vi "ProcessModbusUpdates.vi"(11 "MockHPILCSettings":T1={"ModbusRxDataFIFO"="MockbusPort2RxFIFO", "ModbusTxDataFIFO"="MockbusPort2TxFIFO", "BufferUpdateFIFO"="MockHPILCCommand", "Code17Memory"="MockHPILCCode17", "Code18Memory"="MockHPILCCode18", "Code65Memory"="MockHPILCCode65", "Code66Memory"="MockHPILCCode66", "Code67Memory"="MockHPILCCode67", "Code72Memory"="MockHPILCCode72", "Code80Memory"="MockHPILCCode80", "Code110Memory"="MockHPILCCode110", "CRCDataFIFO"="MockHPILCCRCDataFIFO", "CRCCalculateFIFO"="MockHPILCCRCCalculateFIFO", "CRCFIFO"="MockHPILCCRCFIFO"}) -> ()   [LabVIEW 2016, in "FPGAMockHPILC.lvlib"]
uses:
  FPGAMockHPILC.lvlib
  DataTypes/MockHPILCSettings.ctl
  DataTypes/MockHPModbusUpdateLoopData.ctl
  DataTypes/MockHPModbusUpdateStates.ctl
  <vilib>/Platform/TimedLoop/XDataNode/timing_clust.ctl
  <vilib>/Platform/TimedLoop/XDataNode/nitl_modes.ctl
  <vilib>/Platform/TimedLoop/XDataNode/wakeup.ctl
  <vilib>/rvi/Emulation/niFpgaSctlEmulationGetInTimedLoop.vi
  <vilib>/rvi/Emulation/niFpgaEmulationReportErrorSimple.vi
  <vilib>/rvi/Emulation/niFpgaGetClockAttributes.vi
  <vilib>/rvi/Emulation/niFpgaCriticalErrorInLSC.vi
  <vilib>/rvi/DataTransferAndStorage/Container/Common/niFpgaContainerExecOnDevCompGetState.vi
  <vilib>/rvi/Emulation/niFpgaEmulationIsFPGAContextNoSignature.vi
  <vilib>/rvi/errors/niFpgaSetErrorForExecOnDevCompSimple.vi
  <vilib>/rvi/eio/common/nirviEmuReportErrorAndStop.vi
  <vilib>/rvi/DataTransferAndStorage/Container/Common/niFpgaContainerGetUniqueNameForEmu.vi
  <vilib>/rvi/FIFO/Fifo_Resource/nirvififoEmulationSetSize.vi
  <vilib>/rvi/FIFO/Fifo_Resource/nirviFifoEmulationQueueMgr.vi
  <instcachedir>/0/nirviFifoEmulationQueueMgr_E5CAEC123FF24DC58D834DCA3CDAA9B5.lvgen/nirviFifoEmulationQueueMgr_E5CAEC123FF24DC58D834DCA3CDAA9B5_002.vi
  <vilib>/rvi/FIFO/Fifo_Resource/nirvififoEmulationDetermineInputValidOut.vi
  <vilib>/rvi/FIFO/Fifo_Resource/nirvififoEmulationCreateLock.vi
  <vilib>/rvi/Emulation/niFpgaProcessEmulError.vi
  <vilib>/rvi/FIFO/Fifo_Resource/nirvififoEmulationObtainLock.vi
  <vilib>/rvi/FIFO/Fifo_Resource/nirvififoEmulationReleaseLock.vi
  <vilib>/rvi/occurrence/nirviWaitOnOccurrenceBase.vi
  <vilib>/rvi/errors/nirviReportUnexpectedCaseInternalError.vi
  <vilib>/rvi/errors/nirviReportUnexpectedCaseInternalError (U32).vi
  <vilib>/Utility/error.llb/Clear Errors.vi
  <vilib>/rvi/interface/RandomDataEmulation/niFpgaRandomDataHandleErrors.vi
  <instcachedir>/0/nirviFifoEmulationQueueMgr_E5CAEC123FF24DC58D834DCA3CDAA9B5.lvgen/nirviFifoEmulationQueueMgr_E5CAEC123FF24DC58D834DCA3CDAA9B5_009.vi
  <vilib>/rvi/Memory/Memory_Emulation/niFpgaMemoryEmulationCacheClearOnFirstRun.vi
  <vilib>/rvi/Memory/Memory_Emulation/nirvimemoryEmulationManagerCache_MakeExclusive.vi
  <vilib>/rvi/Memory/Memory_Emulation/niFpgaMemoryEmulationValidateCache.vi
  <vilib>/rvi/Memory/Memory_Emulation/nirvimemoryEmulationManagerCache_InsertValue.vi
  <vilib>/rvi/Memory/Memory_Emulation/nirvimemoryEmulationManagerCache_ReleaseExclusive.vi
  <vilib>/rvi/Memory/Memory_Emulation/nirvimemoryEmulationManagerCache_GetValue.vi
  <vilib>/rvi/Memory/Memory_Emulation/nirvimemoryEmulationManagerCache_SetValue.vi
  <vilib>/rvi/Emulation/niFpgaSctlEmulationResourceMgr.vi
  <instcachedir>/0/nirviFifoEmulationQueueMgr_E5CAEC123FF24DC58D834DCA3CDAA9B5.lvgen/nirviFifoEmulationQueueMgr_E5CAEC123FF24DC58D834DCA3CDAA9B5_004.vi
  <vilib>/Platform/TimedLoop/XDataNode/XDataNode.xnode
  <vilib>/rvi/DataTransferAndStorage/Container/XNode/niFpgaContainer.xnode
  <vilib>/rvi/FIFO/Fifo_Resource/niFpgaFifoEmulationRefIn.vi
  <vilib>/rvi/Memory/Memory_Emulation/niFpgaMemoryEmulationRefIn.vi
  <vilib>/Platform/TimedLoop/XDataNode/XDNodeRunTimeDep.lvlib
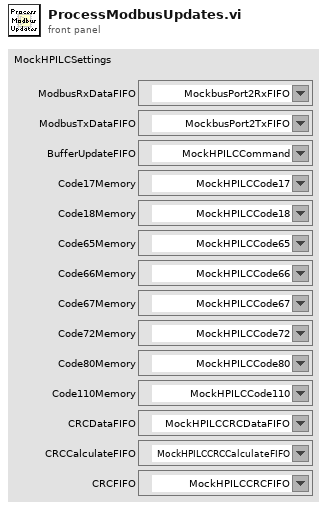
[diagram p1: front panel]
types:
  T1 = typedef "FPGAMockHPILC.lvlib/MockHPILCSettings.ctl" = cluster{"ModbusRxDataFIFO":refnum<k21>, "ModbusTxDataFIFO":refnum<k21>, "BufferUpdateFIFO":refnum<k21>, "Code17Memory":refnum<k21>, "Code18Memory":refnum<k21>, "Code65Memory":refnum<k21>, "Code66Memory":refnum<k21>, "Code67Memory":refnum<k21>, "Code72Memory":refnum<k21>, "Code80Memory":refnum<k21>, "Code110Memory":refnum<k21>, "CRCDataFIFO":refnum<k21>, "CRCCalculateFIFO":refnum<k21>, "CRCFIFO":refnum<k21>}
  T2 = typedef "FPGAMockHPILC.lvlib/MockHPModbusUpdateLoopData.ctl" = cluster{"ModbusUpdateLoopStates":T3, "Address":u8, "Function":u8, "ResponseLength":u8, "ResponseIndex":u8, "Index":u8, "Data":u16, "DelayTicks":u32}
  T3 = typedef "FPGAMockHPILC.lvlib/MockHPModbusUpdateStates.ctl" = enum16{"ReadModbusPort", "ProcessModbusData", "DelayMicroseconds", "WriteAddress", "WriteFunction", "WriteData", "WriteCRCLSB", "WriteCRCMSB", "WriteEndOfFrame", "CalculateCRC"}
  T4 = typedef "XDNodeRunTimeDep.lvlib/timing_clust.ctl" = cluster{"Expected End [f-1]":u64, "Actual End [f-1]":u64, "Finished Late? [f-1]":bool, "Expected End [i-1]":u64, "Actual End [i-1]":u64, "Finished Late? [i-1]":bool, "Expected Start [i]":u64, "Actual Start [i]":u64, "Expected Start [f]":u64, "Actual Start [f]":u64, "Source Name":string, "Structure Name":string, "Period":i64, "Deadline":i64, "Offset":i64, "Start":i64, "Priority":i32, "Timeout":i32, "Mode":T5, "Wakeup Reason":T6, "Error":errorcluster, "Source Type":string, "Secondary Source Type":string, "Global End Time":u64, "Global Start Time":u64, "Frame Duration":u64, "Iteration Duration":u64, "Assigned CPU":i32, "I/O Scan Engine Mode":u32}
  T5 = typedef "XDNodeRunTimeDep.lvlib/nitl_modes.ctl" = enum32{"No Change", "Process missed periods, maintain original phase", "Discard missed periods, maintain original phase", "Process missed periods, ignore original phase", "Discard missed periods, ignore original phase"}
  T6 = typedef "XDNodeRunTimeDep.lvlib/wakeup.ctl" = enum32{"Normal", "Aborted", "Asynchronous wakeup", "Timing source error", "Timed loop error", "Timeout"}
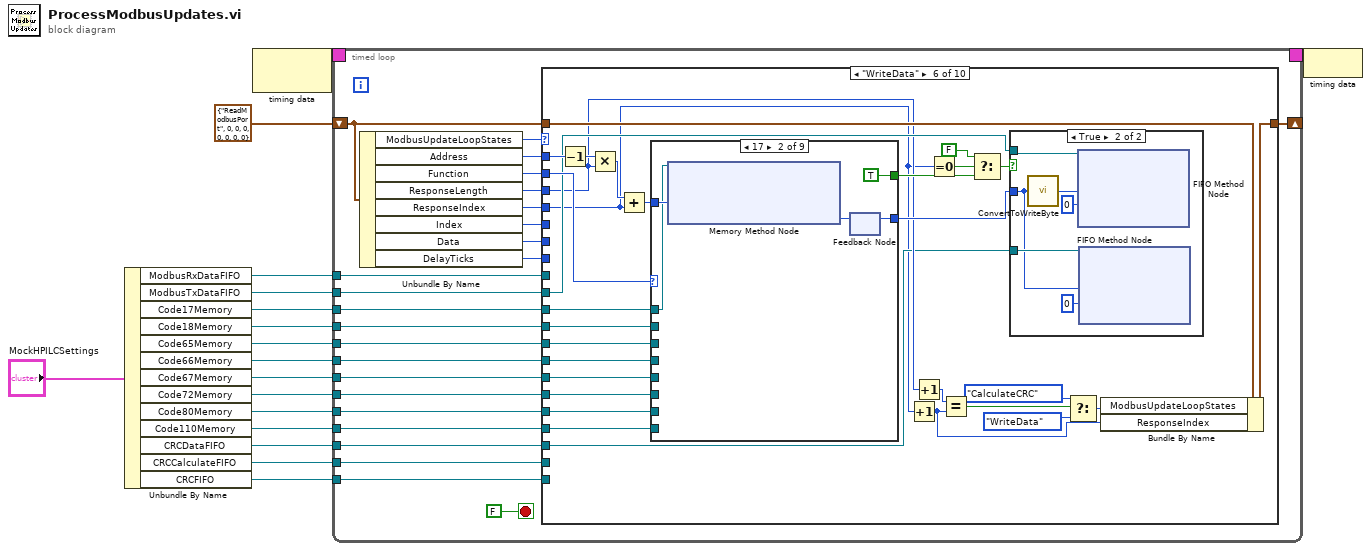
[diagram p0: block diagram]
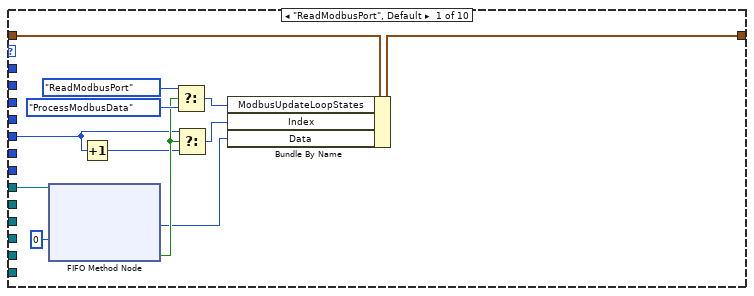
[diagram p2: hidden frame]
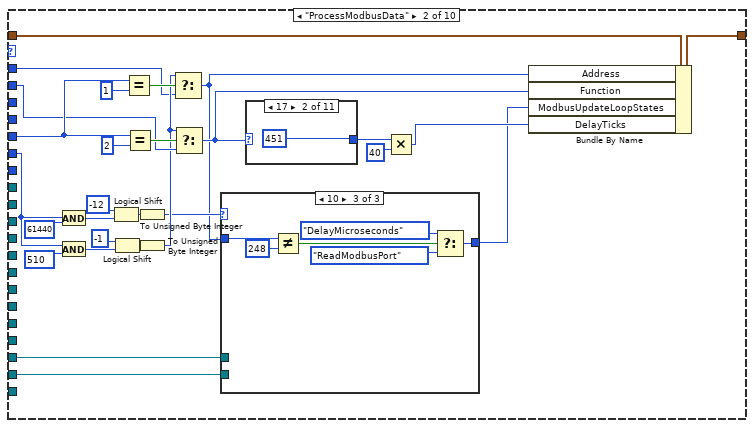
[diagram p3: hidden frame]
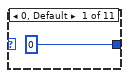
[diagram p4: hidden frame]
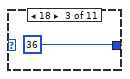
[diagram p5: hidden frame]
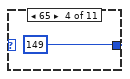
[diagram p6: hidden frame]
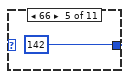
[diagram p7: hidden frame]
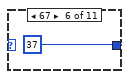
[diagram p8: hidden frame]
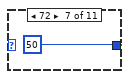
[diagram p9: hidden frame]
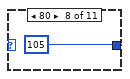
[diagram p10: hidden frame]
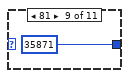
[diagram p11: hidden frame]
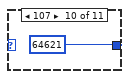
[diagram p12: hidden frame]
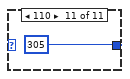
[diagram p13: hidden frame]
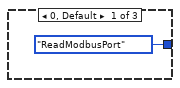
[diagram p14: hidden frame]
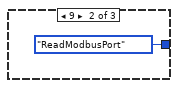
[diagram p15: hidden frame]
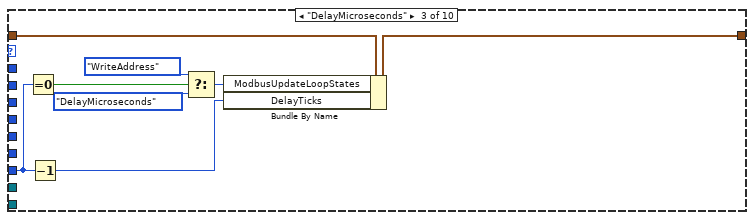
[diagram p16: hidden frame]
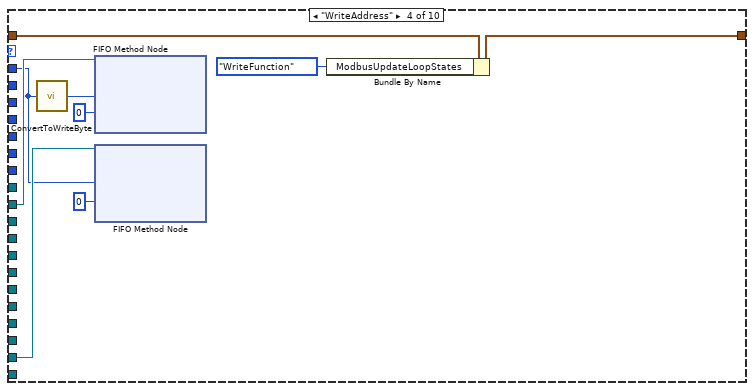
[diagram p17: hidden frame]
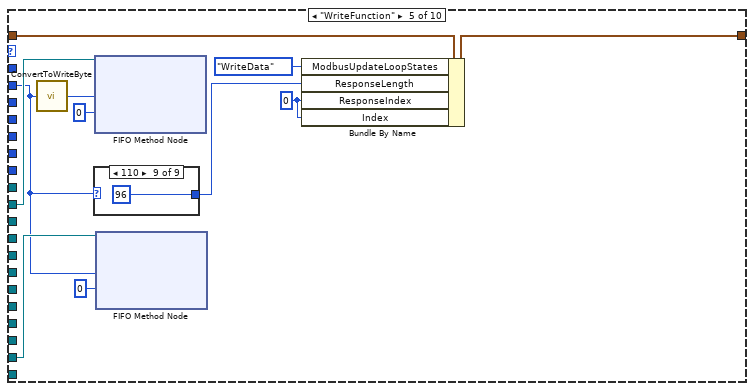
[diagram p18: hidden frame]
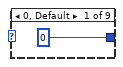
[diagram p19: hidden frame]
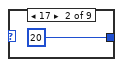
[diagram p20: hidden frame]
diagram:
  n1 = Unbundle By Name("MockHPILCSettings") -> ("ModbusRxDataFIFO"=w13:refnum<k21>, "ModbusTxDataFIFO"=w12:refnum<k21>, "Code17Memory"=w11:refnum<k21>, "Code18Memory"=w10:refnum<k21>, "Code65Memory"=w9:refnum<k21>, "Code66Memory"=w8:refnum<k21>, "Code67Memory"=w7:refnum<k21>, "Code72Memory"=w6:refnum<k21>, "Code80Memory"=w5:refnum<k21>, "Code110Memory"=w4:refnum<k21>, "CRCDataFIFO"=w3:refnum<k21>, "CRCCalculateFIFO"=w2:refnum<k21>, "CRCFIFO"=w1:refnum<k21>)
  n2 = node-c288() -> (w15:T4)  [unwired: 1 in]
  n3 = timed-loop {
    shift-right: [w36] -> _
    shift-left: T2 {"ModbusUpdateLoopStates"=enum."ReadModbusPort", "Address"=0, "Function"=0, "ResponseLength"=0, "ResponseIndex"=0, "Index"=0, "Data"=0, "DelayTicks"=0} ("MockHPBufferUpdateLoopData") -> [w35]
    timing: w15 -> [_]
    timing-out: [_] -> w14
    tunnel: w13 -> [w34]
    tunnel: w12 -> [w30]
    tunnel: w11 -> [w29]
    tunnel: w10 -> [w28]
    tunnel: w9 -> [w27]
    tunnel: w8 -> [w26]
    tunnel: w7 -> [w25]
    tunnel: w6 -> [w24]
    tunnel: w5 -> [w23]
    tunnel: w4 -> [w22]
    tunnel: w3 -> [w21]
    tunnel: w2 -> [w20]
    tunnel: w1 -> [w19]
    stop <- FALSE stop-if-true
    n4 = Unbundle By Name(w35) -> ("ModbusUpdateLoopStates"=w41:T3, "Address"=w40:u8, "Function"=w39:u8, "ResponseLength"=w38:u8, "ResponseIndex"=w37:u8, "Index"=w33:u8, "Data"=w32:u16, "DelayTicks"=w18:u32)
    n5 = case shown="\"WriteData\"" w41 {
      tunnel: w40 -> [_ w56 _ w110 _ w162 _ _ _ _]
      tunnel: w39 -> [_ w65 _ _ w119 w165 _ _ _ _]
      tunnel: w38 -> [_ _ _ _ _ w141 _ _ _ _]
      tunnel: w37 -> [_ _ _ _ _ w138 _ _ _ _]
      tunnel: [w42 w80 w107 w112 w123 w166 w217 w228 w242 w250] -> w36
      tunnel: w35 -> [w43 w81 w108 w114 w125 w167 w221 w229 w243 w255]
      tunnel: w34 -> [w53 _ _ _ _ _ _ _ _ _]
      tunnel: w33 -> [w47 w66 _ _ _ _ _ _ _ _]
      tunnel: w32 -> [_ w73 _ _ _ _ _ _ _ _]
      tunnel: w30 -> [_ _ _ w117 w128 w158 _ w223 w237 w254]
      tunnel: w29 -> [_ _ _ _ _ w164 _ _ _ _]
      tunnel: w28 -> [_ _ _ _ _ w157 _ _ _ _]
      tunnel: w27 -> [_ _ _ _ _ w156 _ _ _ _]
      tunnel: w26 -> [_ _ _ _ _ w155 _ _ _ _]
      tunnel: w25 -> [_ _ _ _ _ w154 _ _ _ _]
      tunnel: w24 -> [_ _ _ _ _ w153 _ _ _ _]
      tunnel: w23 -> [_ _ _ _ _ w152 _ _ _ _]
      tunnel: w22 -> [_ _ _ _ _ w151 _ _ _ _]
      tunnel: w21 -> [_ w70 _ w111 w120 w139 _ _ _ _]
      tunnel: w20 -> [_ w69 _ _ _ _ w220 _ _ _]
      tunnel: w19 -> [_ _ _ _ _ _ _ w227 w241 _]
      tunnel: w18 -> [_ _ w102 _ _ _ _ _ _ _]
      frame "ReadModbusPort", Default {
        n6 = xnode ("FIFO Method Node")("Timeout"=0, "FIFO In"=w53) -> ("Element"=w44:u16, "Timed Out?"=w49:bool)  [unwired: 1 out]
        n7 = Increment(x=w47) -> (x+1=w48:u8)
        n8 = Select(t=MockHPModbusUpdateStates."ReadModbusPort", s=w49, f=MockHPModbusUpdateStates."ProcessModbusData") -> (s? t:f=w46:T3)
        n9 = Select(t=w47, s=w49, f=w48) -> (s? t:f=w45:u8)
        n10 = Bundle By Name(cluster=w43, "ModbusUpdateLoopStates"=w46, "Index"=w45, "Data"=w44) -> (w42:T2)
      }
      frame "ProcessModbusData" {
        n11 = And(x=w73, y=u16 61440) -> (x .and. y?=w75:u16)
        n12 = And(x=w73, y=u16 510) -> (x .and. y?=w78:u16)
        n13 = Logical Shift(y=i16 -12, x=w75) -> (x << y=w62:u16)
        n14 = Logical Shift(y=i16 -1, x=w78) -> (x << y=w64:u16)
        n15 = Equal?(x=w66, y=u8 1) -> (x = y?=w71:bool)
        n16 = Equal?(x=w66, y=u8 2) -> (x = y?=w68:bool)
        n17 = To Unsigned Byte Integer(number=w62) -> (unsigned 8bit integer=w61:u8)
        n18 = To Unsigned Byte Integer(number=w64) -> (unsigned 8bit integer=w63:u8)
        n19 = Select(t=w63, s=w71, f=w56) -> (s? t:f=w55:u8)
        n20 = Select(t=w63, s=w68, f=w65) -> (s? t:f=w60:u8)
        n21 = case shown="10" w61 {
          tunnel: w70 -> [_ _ _]
          tunnel: w69 -> [_ _ _]
          tunnel: [MockHPModbusUpdateStates."ReadModbusPort" ("f") MockHPModbusUpdateStates."ReadModbusPort" ("f") w100] -> w54
          tunnel: w55 -> [_ _ w96]
          frame 0, Default {
          }
          frame 9 {
          }
          frame 10 {
            n22 = Not Equal?(x=w96, y=u8 248) -> (x != y?=w95:bool)
            n23 = Select(t=MockHPModbusUpdateStates."DelayMicroseconds" ("f"), s=w95, f=MockHPModbusUpdateStates."ReadModbusPort") -> (s? t:f=w100:T3)
          }
        }
        n24 = case shown="17" w60 {
          tunnel: [u32 0 ("Count(uSec)") u32 451 ("Count(uSec)") u32 36 ("Count(uSec)") u32 149 ("Count(uSec)") u32 142 ("Count(uSec)") u32 37 ("Count(uSec)") u32 50 ("Count(uSec)") u32 105 ("Count(uSec)") u32 35871 ("Count(uSec)") u32 64621 ("Count(uSec)") u32 305 ("Count(uSec)")] -> w59
          frame 0, Default {
          }
          frame 17 {
          }
          frame 18 {
          }
          frame 65 {
          }
          frame 66 {
          }
          frame 67 {
          }
          frame 72 {
          }
          frame 80 {
          }
          frame 81 {
          }
          frame 107 {
          }
          frame 110 {
          }
        }
        n25 = Multiply(x=w59, y=u32 40) -> (x*y=w57:u32)
        n26 = Bundle By Name(cluster=w81, "Address"=w55, "Function"=w60, "ModbusUpdateLoopStates"=w54, "DelayTicks"=w57) -> (w80:T2)
      }
      frame "DelayMicroseconds" {
        n27 = Equal To 0?(x=w102) -> (x = 0?=w106:bool)
        n28 = Decrement(x=w102) -> (x-1=w101:u32)
        n29 = Select(t=MockHPModbusUpdateStates."WriteAddress", s=w106, f=MockHPModbusUpdateStates."DelayMicroseconds") -> (s? t:f=w105:T3)
        n30 = Bundle By Name(cluster=w108, "ModbusUpdateLoopStates"=w105, "DelayTicks"=w101) -> (w107:T2)
      }
      frame "WriteAddress" {
        n31 = call "ConvertToWriteByte.vi"("Input"=w110) -> ("Output"=w116:u16)
        n32 = xnode ("FIFO Method Node")("Element"=w116, "Timeout"=0, "FIFO In"=w117) -> ()  [unwired: 2 out]
        n33 = xnode ("FIFO Method Node")("Element"=w110, "Timeout"=0, "FIFO In"=w111) -> ()  [unwired: 2 out]
        n34 = Bundle By Name(cluster=w114, "ModbusUpdateLoopStates"=MockHPModbusUpdateStates."WriteFunction") -> (w112:T2)
      }
      frame "WriteFunction" {
        w121 = u8 0 ("ResponseIndex")
        n35 = call "ConvertToWriteByte.vi"("Input"=w119) -> ("Output"=w127:u16)
        n36 = case shown="110" w119 {
          tunnel: [u8 0 ("ResponseLength") u8 20 ("ResponseLength") u8 5 ("ResponseLength") u8 2 ("ResponseLength") u8 9 ("ResponseLength") u8 9 ("ResponseLength") u8 1 ("ResponseLength") u8 1 ("ResponseLength") u8 96 ("ResponseLength")] -> w122
          frame 0, Default {
          }
          frame 17 {
          }
          frame 18 {
          }
          frame 65 {
          }
          frame 66 {
          }
          frame 67 {
          }
          frame 72 {
          }
          frame 80 {
          }
          frame 110 {
          }
        }
        n37 = xnode ("FIFO Method Node")("Element"=w127, "Timeout"=0, "FIFO In"=w128) -> ()  [unwired: 2 out]
        n38 = xnode ("FIFO Method Node")("Element"=w119, "Timeout"=0, "FIFO In"=w120) -> ()  [unwired: 2 out]
        n39 = Bundle By Name(cluster=w125, "ModbusUpdateLoopStates"=MockHPModbusUpdateStates."WriteData", "ResponseLength"=w122, "ResponseIndex"=w121, "Index"=w121) -> (w123:T2)
      }
      frame "WriteData" {
        n40 = Decrement(x=w162) -> (x-1=w163:u8)
        n41 = Multiply(x=w163, y=w141) -> (x*y=w161:u8)
        n42 = Add(x=w161, y=w138) -> (x+y=w160:u8)
        n43 = case shown="17" w165 {
          tunnel: w164 -> [_ w176 _ _ _ _ _ _ _]
          tunnel: w160 -> [_ w180 w185 w190 w195 w200 w205 w210 w215]
          tunnel: [u8 0 ("Data") w177 w182 w187 w192 w197 w202 w207 w212] -> w159
          tunnel: [FALSE TRUE TRUE TRUE TRUE TRUE TRUE TRUE TRUE] -> w144
          tunnel: w157 -> [_ _ w181 _ _ _ _ _ _]
          tunnel: w156 -> [_ _ _ w186 _ _ _ _ _]
          tunnel: w155 -> [_ _ _ _ w191 _ _ _ _]
          tunnel: w154 -> [_ _ _ _ _ w196 _ _ _]
          tunnel: w153 -> [_ _ _ _ _ _ w201 _ _]
          tunnel: w152 -> [_ _ _ _ _ _ _ w206 _]
          tunnel: w151 -> [_ _ _ _ _ _ _ _ w211]
          frame 0, Default {
          }
          frame 17 {
            n44 = xnode ("Memory Method Node")("Address"=w180, "Memory In"=w176) -> ("Data"=w178:u8)  [unwired: 1 out]
            n45 = feedback-in #1(w178) -> ()
            n46 = feedback #1() -> (w177:u8)  [unwired: 1 in]
          }
          frame 18 {
            n47 = xnode ("Memory Method Node")("Address"=w185, "Memory In"=w181) -> ("Data"=w183:u8)  [unwired: 1 out]
            n48 = feedback-in #2(w183) -> ()
            n49 = feedback #2() -> (w182:u8)  [unwired: 1 in]
          }
          frame 65 {
            n50 = xnode ("Memory Method Node")("Address"=w190, "Memory In"=w186) -> ("Data"=w188:u8)  [unwired: 1 out]
            n51 = feedback-in #3(w188) -> ()
            n52 = feedback #3() -> (w187:u8)  [unwired: 1 in]
          }
          frame 66 {
            n53 = xnode ("Memory Method Node")("Address"=w195, "Memory In"=w191) -> ("Data"=w193:u8)  [unwired: 1 out]
            n54 = feedback-in #4(w193) -> ()
            n55 = feedback #4() -> (w192:u8)  [unwired: 1 in]
          }
          frame 67 {
            n56 = xnode ("Memory Method Node")("Address"=w200, "Memory In"=w196) -> ("Data"=w198:u8)  [unwired: 1 out]
            n57 = feedback-in #5(w198) -> ()
            n58 = feedback #5() -> (w197:u8)  [unwired: 1 in]
          }
          frame 72 {
            n59 = xnode ("Memory Method Node")("Address"=w205, "Memory In"=w201) -> ("Data"=w203:u8)  [unwired: 1 out]
            n60 = feedback-in #6(w203) -> ()
            n61 = feedback #6() -> (w202:u8)  [unwired: 1 in]
          }
          frame 80 {
            n62 = xnode ("Memory Method Node")("Address"=w210, "Memory In"=w206) -> ("Data"=w208:u8)  [unwired: 1 out]
            n63 = feedback-in #7(w208) -> ()
            n64 = feedback #7() -> (w207:u8)  [unwired: 1 in]
          }
          frame 110 {
            n65 = xnode ("Memory Method Node")("Address"=w215, "Memory In"=w211) -> ("Data"=w213:u8)  [unwired: 1 out]
            n66 = feedback-in #8(w213) -> ()
            n67 = feedback #8() -> (w212:u8)  [unwired: 1 in]
          }
        }
        n68 = Increment(x=w138) -> (x+1=w146:u8)
        n69 = Increment(x=w141) -> (x+1=w140:u8)
        n70 = Equal To 0?(x=w138) -> (x = 0?=w145:bool)
        n71 = Equal?(x=w140, y=w146) -> (x = y?=w150:bool)
        n72 = Select(t=FALSE, s=w145, f=w144) -> (s? t:f=w143:bool)
        n73 = case shown="True" w143 {
          tunnel: w159 -> [_ w169]
          tunnel: w158 -> [_ w171]
          tunnel: w139 -> [_ w170]
          frame False {
          }
          frame True {
            n74 = call "ConvertToWriteByte.vi"("Input"=w169) -> ("Output"=w172:u16)
            n75 = xnode ("FIFO Method Node")("Element"=w172, "Timeout"=0, "FIFO In"=w171) -> ()  [unwired: 2 out]
            n76 = xnode ("FIFO Method Node")("Element"=w169, "Timeout"=0, "FIFO In"=w170) -> ()  [unwired: 2 out]
          }
        }
        n77 = Select(t=MockHPModbusUpdateStates."CalculateCRC", s=w150, f=MockHPModbusUpdateStates."WriteData") -> (s? t:f=w147:T3)
        n78 = Bundle By Name(cluster=w167, "ModbusUpdateLoopStates"=w147, "ResponseIndex"=w146) -> (w166:T2)
      }
      frame "CalculateCRC" {
        n79 = xnode "FIFO Write"("Element"=TRUE, "Timeout"=0, "FIFO In"=w220) -> ()  [unwired: 2 out]
        n80 = Bundle By Name(cluster=w221, "ModbusUpdateLoopStates"=MockHPModbusUpdateStates."WriteCRCLSB") -> (w217:T2)
      }
      frame "WriteCRCLSB" {
        n81 = xnode ("FIFO Read")("Timeout"=0, "FIFO In"=w227) -> ("Element"=w224:u8, "Timed Out?"=w225:bool)  [unwired: 1 out]
        n82 = case shown="False" w225 {
          tunnel: w224 -> [w234 _]
          tunnel: w223 -> [w233 _]
          tunnel: [MockHPModbusUpdateStates."WriteCRCMSB" ("ModbusUpdateLoopStates") MockHPModbusUpdateStates."WriteCRCLSB" ("ModbusUpdateLoopStates")] -> w222
          frame False {
            n83 = call "ConvertToWriteByte.vi"("Input"=w234) -> ("Output"=w232:u16)
            n84 = xnode ("FIFO Write")("Element"=w232, "Timeout"=0, "FIFO In"=w233) -> ()  [unwired: 2 out]
          }
          frame True {
          }
        }
        n85 = Bundle By Name(cluster=w229, "ModbusUpdateLoopStates"=w222) -> (w228:T2)
      }
      frame "WriteCRCMSB" {
        n86 = xnode ("FIFO Read")("Timeout"=0, "FIFO In"=w241) -> ("Element"=w238:u8, "Timed Out?"=w239:bool)  [unwired: 1 out]
        n87 = case shown="False" w239 {
          tunnel: w238 -> [w248 _]
          tunnel: w237 -> [w247 _]
          tunnel: [MockHPModbusUpdateStates."WriteEndOfFrame" ("ModbusUpdateLoopStates") MockHPModbusUpdateStates."WriteCRCMSB" ("ModbusUpdateLoopStates")] -> w236
          frame False {
            n88 = call "ConvertToWriteByte.vi"("Input"=w248) -> ("Output"=w246:u16)
            n89 = xnode ("FIFO Write")("Element"=w246, "Timeout"=0, "FIFO In"=w247) -> ()  [unwired: 2 out]
          }
          frame True {
          }
        }
        n90 = Bundle By Name(cluster=w243, "ModbusUpdateLoopStates"=w236) -> (w242:T2)
      }
      frame "WriteEndOfFrame" {
        n91 = xnode ("FIFO Write")("Element"=u16 8416, "Timeout"=0, "FIFO In"=w254) -> ()  [unwired: 2 out]
        n92 = Bundle By Name(cluster=w255, "ModbusUpdateLoopStates"=MockHPModbusUpdateStates."ReadModbusPort") -> (w250:T2)
      }
    }
  }
  n93 = node-c288(w14) -> ()
